vi "S4GUI_001.vi"() -> ()   [LabVIEW 2018] (continued)
        n876 = call-dynamic "Write PREV_FT.vi"("error in (no error)"=w1779, "PREV_FT"=w1776, "Interface in"=w1780) -> ("error out"=w1777:errorcluster, "Interface out"=w1778:refnum<class "Interface.lvclass">)  [unwired: 7 in]
        n877 = call-dynamic "Get CCD_Config.vi"("error in (no error)"=w1777, "Interface in"=w1778) -> ("error out"=w1817:errorcluster, "output cluster"=w1819:T24, "Interface out"=w1818:refnum<class "Interface.lvclass">)  [unwired: 7 in]
        n878 = Bundle By Name(cluster=w1819, "INITIAL_LINE"=w1816, "INITIAL_COLUMN"=w1815, "FINAL_LINE"=w1814, "FINAL_COLUMN"=w1813, "VBIN"=w1812, "HBIN"=w1811, "PREAMP"=w1810, "EM_GAIN"=w1809, "READOUT_RATE"=w1808, "SHUTTER_OPENING_TIME"=w1807, "SHUTTER_CLOSING_TIME"=w1806, "VERTICAL_SHIFT_SPEED"=w1805, "READ_MODE"=w1804, "VERTICAL_CLOCK_VOLTAGE"=w1803, "AD_CHANNEL"=w1802, "SHUTTER_MODE"=w1801, "SHUTTER_TTL"=w1800, "TRIGGER_MODE"=w1799, "FRAME_TRANSFER"=w1776, "ACQUISITION_MODE"=w1798, "EM_MODE"=w1797) -> (w1787:T24)
        n879 = call-dynamic "Set CCD_Config.vi"("error in (no error)"=w1817, "input cluster"=w1787, "Interface in"=w1818) -> ("error out"=w1822:errorcluster, "Interface out"=w1823:refnum<class "Interface.lvclass">)  [unwired: 7 in]
        n880 = Flatten To String(anything=w1787, error in (no error)=w1822) -> (data string=w1825:string, error out=w1824:errorcluster)  [unwired: 2 in, 1 out]
        n881 = call "Write flatted cluster.vi"("error in (no error)"=w1824, "flatted cluster"=w1825, "Interface in"=w1823) -> ("error out"=w1821:errorcluster, "Interface out"=w1820:refnum<class "Interface.lvclass">)  [unwired: 7 in]
        n882 = call-dynamic "Write Interface.vi"("error in (no error)"=w1821, "Interface.lvclass"=w1820, "Channel in"=w1838) -> ("error out"=w1792:errorcluster, "Channel out"=w1795:refnum<class "Channel.lvclass">)  [unwired: 7 in]
        n883 = call "Write section_name.vi"("error in (no error)"=w1792, "section_name"="CCD_ACS4", "Channel in"=w1795) -> ("error out"=w1791:errorcluster, "Channel out"=w1794:refnum<class "Channel.lvclass">)  [unwired: 7 in]
        n884 = call-dynamic "save config.vi"("error in (no error)"=w1791, "file config"="lastsaved.cfg", "Channel in"=w1794) -> ("error out"=w1790:errorcluster, "Channel out"=w1793:refnum<class "Channel.lvclass">)  [unwired: 7 in]
        n885 = call-dynamic "Read State Machine.vi"("error in (no error)"=w1790, "Device in"=w1793) -> ("error out"=w1832:errorcluster, "State Machine.lvclass"=w1834:refnum<class "State Machine.lvclass">, "Device out"=w1835:refnum<class "Channel.lvclass">)  [unwired: 7 in]
        n886 = call-dynamic "Write State.vi"("error in (no error)"=w1832, "State"=60, "State Machine in"=w1834) -> ("error out"=w1831:errorcluster, "State Machine out"=w1833:refnum<class "State Machine.lvclass">)  [unwired: 7 in]
        n887 = call-dynamic "Write State Machine.vi"("error in (no error)"=w1831, "State Machine.lvclass"=w1833, "Device in"=w1835) -> ("error out"=w1828:errorcluster, "Device out"=w1829:refnum<class "Channel.lvclass">)  [unwired: 7 in]
        n888 = call-dynamic "Write Channel.vi"("error in (no error)"=w1828, "Channel.lvclass"=w1829, "Acquisition in"=w1840) -> ("error out"=w1827:errorcluster, "Acquisition out"=w1826:refnum<class "Acquisition.lvclass">)  [unwired: 7 in]
        n889 = call-dynamic "Write AcquisitionD.vi"("error in (no error)"=w1827, "Acquisition.lvclass"=w1826, "S4ACS_GUI in"=w1842) -> ("error out"=w1781:errorcluster, "S4ACS_GUI out"=w1782:refnum<class "S4GUI.lvclass">)  [unwired: 7 in]
        n890 = call "Write cfg file.vi"("error in (no error)"=w1781, "cfg file"="lastsaved.cfg", "S4ACS_GUI in"=w1782) -> ("error out"=w1784:errorcluster, "S4ACS_GUI out"=w1785:refnum<class "S4GUI.lvclass">)  [unwired: 7 in]
      }
      event "Restore Default ch1": Value Change {
        n891 = event-data() -> ()  [unwired: 1 in, 6 out]
        n892 = call-dynamic "Read AcquisitionA.vi"("error in (no error)"=w1875, "S4ACS_GUI in"=w1876) -> ("error out"=w1871:errorcluster, "Acquisition.lvclass"=w1873:refnum<class "Acquisition.lvclass">, "S4ACS_GUI out"=w1874:refnum<class "S4GUI.lvclass">)  [unwired: 7 in]
        n893 = call-dynamic "Read Channel.vi"("error in (no error)"=w1871, "Acquisition in"=w1873) -> ("error out"=w1858:errorcluster, "Channel.lvclass"=w1860:refnum<class "Channel.lvclass">, "Acquisition out"=w1872:refnum<class "Acquisition.lvclass">)  [unwired: 7 in]
        n894 = call "Write section_name.vi"("error in (no error)"=w1858, "section_name"="CCD_ACS1", "Channel in"=w1860) -> ("error out"=w1857:errorcluster, "Channel out"=w1859:refnum<class "Channel.lvclass">)  [unwired: 7 in]
        n895 = call-dynamic "load config.vi"("error in (no error)"=w1857, "cfg file name"="default.cfg", "Channel in"=w1859) -> ("error out"=w1855:errorcluster, "Channel out"=w1856:refnum<class "Channel.lvclass">)  [unwired: 7 in]
        n896 = call-dynamic "Read State Machine.vi"("error in (no error)"=w1855, "Device in"=w1856) -> ("error out"=w1867:errorcluster, "State Machine.lvclass"=w1869:refnum<class "State Machine.lvclass">, "Device out"=w1870:refnum<class "Channel.lvclass">)  [unwired: 7 in]
        n897 = call-dynamic "Write State.vi"("error in (no error)"=w1867, "State"=60, "State Machine in"=w1869) -> ("error out"=w1866:errorcluster, "State Machine out"=w1868:refnum<class "State Machine.lvclass">)  [unwired: 7 in]
        n898 = call-dynamic "Write State Machine.vi"("error in (no error)"=w1866, "State Machine.lvclass"=w1868, "Device in"=w1870) -> ("error out"=w1851:errorcluster, "Device out"=w1847:refnum<class "Channel.lvclass">)  [unwired: 7 in]
        n899 = call "Write section_name.vi"("error in (no error)"=w1851, "section_name"="CCD_ACS1", "Channel in"=w1847) -> ("error out"=w1852:errorcluster, "Channel out"=w1846:refnum<class "Channel.lvclass">)  [unwired: 7 in]
        n900 = call-dynamic "save config.vi"("error in (no error)"=w1852, "file config"="lastsaved.cfg", "Channel in"=w1846) -> ("error out"=w1850:errorcluster, "Channel out"=w1845:refnum<class "Channel.lvclass">)  [unwired: 7 in]
        n901 = call-dynamic "Write Channel.vi"("error in (no error)"=w1850, "Channel.lvclass"=w1845, "Acquisition in"=w1872) -> ("error out"=w1864:errorcluster, "Acquisition out"=w1863:refnum<class "Acquisition.lvclass">)  [unwired: 7 in]
        n902 = call-dynamic "Write AcquisitionA.vi"("error in (no error)"=w1864, "Acquisition.lvclass"=w1863, "S4ACS_GUI in"=w1874) -> ("error out"=w1862:errorcluster, "S4ACS_GUI out"=w1853:refnum<class "S4GUI.lvclass">)  [unwired: 7 in]
      }
      event "Load Button": Value Change {
        n903 = event-data() -> ()  [unwired: 1 in, 6 out]
        n904 = call <vilib>:"Application Directory.vi"() -> ("Application Directory"=w1888:path)
        n905 = call "File Dialog"("start path"=w1888, "prompt"="Select file...", "button label"="Open", "default name"="lastsaved.cfg", "error in"=w1882, "pattern (all files)"="*.cfg") -> ("selected path"=w1880:path, "cancelled"=w1883:bool, "error out"=→"error out 2":errorcluster)  [unwired: 6 in, 1 out]
        "selected path" <- w1880
        n906 = Path To String(path=w1880) -> (string=w1879:string)
        n907 = Match Pattern(string=w1879, regular expression="SPARC4_GUI\\") -> (after substring=w1877:string)  [unwired: 1 in, 3 out]
        n908 = case shown="False" w1883 {
          tunnel: w1891 -> [w2000 w2002]
          tunnel: [w1916 w2002] -> w1890
          tunnel: [w1914 w2001] -> w1889
          tunnel: w1882 -> [w1913 w2001]
          tunnel: w1877 -> [w1912 _]
          frame False {
            n909 = call-dynamic "Read AcquisitionA.vi"("error in (no error)"=w1913, "S4ACS_GUI in"=w2000) -> ("error out"=w1996:errorcluster, "Acquisition.lvclass"=w1998:refnum<class "Acquisition.lvclass">, "S4ACS_GUI out"=w1999:refnum<class "S4GUI.lvclass">)  [unwired: 7 in]
            n910 = call-dynamic "Read Channel.vi"("error in (no error)"=w1996, "Acquisition in"=w1998) -> ("error out"=w1983:errorcluster, "Channel.lvclass"=w1985:refnum<class "Channel.lvclass">, "Acquisition out"=w1997:refnum<class "Acquisition.lvclass">)  [unwired: 7 in]
            n911 = call "Write section_name.vi"("error in (no error)"=w1983, "section_name"="CCD_ACS1", "Channel in"=w1985) -> ("error out"=w1982:errorcluster, "Channel out"=w1984:refnum<class "Channel.lvclass">)  [unwired: 7 in]
            n912 = call-dynamic "load config.vi"("error in (no error)"=w1982, "cfg file name"=w1912, "Channel in"=w1984) -> ("error out"=w1908:errorcluster, "Channel out"=w1910:refnum<class "Channel.lvclass">)  [unwired: 7 in]
            n913 = call-dynamic "save config.vi"("error in (no error)"=w1908, "file config"="lastsaved.cfg", "Channel in"=w1910) -> ("error out"=w1911:errorcluster, "Channel out"=w1909:refnum<class "Channel.lvclass">)  [unwired: 7 in]
            n914 = call-dynamic "Read State Machine.vi"("error in (no error)"=w1911, "Device in"=w1909) -> ("error out"=w1992:errorcluster, "State Machine.lvclass"=w1994:refnum<class "State Machine.lvclass">, "Device out"=w1995:refnum<class "Channel.lvclass">)  [unwired: 7 in]
            n915 = call-dynamic "Write State.vi"("error in (no error)"=w1992, "State"=60, "State Machine in"=w1994) -> ("error out"=w1991:errorcluster, "State Machine out"=w1993:refnum<class "State Machine.lvclass">)  [unwired: 7 in]
            n916 = call-dynamic "Write State Machine.vi"("error in (no error)"=w1991, "State Machine.lvclass"=w1993, "Device in"=w1995) -> ("error out"=w1988:errorcluster, "Device out"=w1989:refnum<class "Channel.lvclass">)  [unwired: 7 in]
            n917 = call-dynamic "Write Channel.vi"("error in (no error)"=w1988, "Channel.lvclass"=w1989, "Acquisition in"=w1997) -> ("error out"=w1987:errorcluster, "Acquisition out"=w1986:refnum<class "Acquisition.lvclass">)  [unwired: 7 in]
            n918 = call-dynamic "Write AcquisitionA.vi"("error in (no error)"=w1987, "Acquisition.lvclass"=w1986, "S4ACS_GUI in"=w1999) -> ("error out"=w1923:errorcluster, "S4ACS_GUI out"=w1922:refnum<class "S4GUI.lvclass">)  [unwired: 7 in]
            n919 = call "Read AcquisitionB.vi"("error in (no error)"=w1923, "S4ACS_GUI in"=w1922) -> ("error out"=w1965:errorcluster, "Acquisition.lvclass"=w1963:refnum<class "Acquisition.lvclass">, "S4ACS_GUI out"=w1962:refnum<class "S4GUI.lvclass">)  [unwired: 7 in]
            n920 = call-dynamic "Read Channel.vi"("error in (no error)"=w1965, "Acquisition in"=w1963) -> ("error out"=w1978:errorcluster, "Channel.lvclass"=w1976:refnum<class "Channel.lvclass">, "Acquisition out"=w1964:refnum<class "Acquisition.lvclass">)  [unwired: 7 in]
            n921 = call "Write section_name.vi"("error in (no error)"=w1978, "section_name"="CCD_ACS2", "Channel in"=w1976) -> ("error out"=w1979:errorcluster, "Channel out"=w1977:refnum<class "Channel.lvclass">)  [unwired: 7 in]
            n922 = call-dynamic "load config.vi"("error in (no error)"=w1979, "cfg file name"=w1912, "Channel in"=w1977) -> ("error out"=w1905:errorcluster, "Channel out"=w1903:refnum<class "Channel.lvclass">)  [unwired: 7 in]
            n923 = call-dynamic "save config.vi"("error in (no error)"=w1905, "file config"="lastsaved.cfg", "Channel in"=w1903) -> ("error out"=w1904:errorcluster, "Channel out"=w1902:refnum<class "Channel.lvclass">)  [unwired: 7 in]
            n924 = call-dynamic "Read State Machine.vi"("error in (no error)"=w1904, "Device in"=w1902) -> ("error out"=w1969:errorcluster, "State Machine.lvclass"=w1967:refnum<class "State Machine.lvclass">, "Device out"=w1966:refnum<class "Channel.lvclass">)  [unwired: 7 in]
            n925 = call-dynamic "Write State.vi"("error in (no error)"=w1969, "State"=60, "State Machine in"=w1967) -> ("error out"=w1970:errorcluster, "State Machine out"=w1968:refnum<class "State Machine.lvclass">)  [unwired: 7 in]
            n926 = call-dynamic "Write State Machine.vi"("error in (no error)"=w1970, "State Machine.lvclass"=w1968, "Device in"=w1966) -> ("error out"=w1973:errorcluster, "Device out"=w1972:refnum<class "Channel.lvclass">)  [unwired: 7 in]
            n927 = call-dynamic "Write Channel.vi"("error in (no error)"=w1973, "Channel.lvclass"=w1972, "Acquisition in"=w1964) -> ("error out"=w1974:errorcluster, "Acquisition out"=w1975:refnum<class "Acquisition.lvclass">)  [unwired: 7 in]
            n928 = call "Write AcquisitionB.vi"("error in (no error)"=w1974, "Acquisition.lvclass"=w1975, "S4ACS_GUI in"=w1962) -> ("error out"=w1921:errorcluster, "S4ACS_GUI out"=w1920:refnum<class "S4GUI.lvclass">)  [unwired: 7 in]
            n929 = call-dynamic "Read AcquisitionC.vi"("error in (no error)"=w1921, "S4ACS_GUI in"=w1920) -> ("error out"=w1958:errorcluster, "Acquisition.lvclass"=w1960:refnum<class "Acquisition.lvclass">, "S4ACS_GUI out"=w1961:refnum<class "S4GUI.lvclass">)  [unwired: 7 in]
            n930 = call-dynamic "Read Channel.vi"("error in (no error)"=w1958, "Acquisition in"=w1960) -> ("error out"=w1945:errorcluster, "Channel.lvclass"=w1947:refnum<class "Channel.lvclass">, "Acquisition out"=w1959:refnum<class "Acquisition.lvclass">)  [unwired: 7 in]
            n931 = call "Write section_name.vi"("error in (no error)"=w1945, "section_name"="CCD_ACS3", "Channel in"=w1947) -> ("error out"=w1944:errorcluster, "Channel out"=w1946:refnum<class "Channel.lvclass">)  [unwired: 7 in]
            n932 = call-dynamic "load config.vi"("error in (no error)"=w1944, "cfg file name"=w1912, "Channel in"=w1946) -> ("error out"=w1900:errorcluster, "Channel out"=w1898:refnum<class "Channel.lvclass">)  [unwired: 7 in]
            n933 = call-dynamic "save config.vi"("error in (no error)"=w1900, "file config"="lastsaved.cfg", "Channel in"=w1898) -> ("error out"=w1899:errorcluster, "Channel out"=w1897:refnum<class "Channel.lvclass">)  [unwired: 7 in]
            n934 = call-dynamic "Read State Machine.vi"("error in (no error)"=w1899, "Device in"=w1897) -> ("error out"=w1954:errorcluster, "State Machine.lvclass"=w1956:refnum<class "State Machine.lvclass">, "Device out"=w1957:refnum<class "Channel.lvclass">)  [unwired: 7 in]
            n935 = call-dynamic "Write State.vi"("error in (no error)"=w1954, "State"=60, "State Machine in"=w1956) -> ("error out"=w1953:errorcluster, "State Machine out"=w1955:refnum<class "State Machine.lvclass">)  [unwired: 7 in]
            n936 = call-dynamic "Write State Machine.vi"("error in (no error)"=w1953, "State Machine.lvclass"=w1955, "Device in"=w1957) -> ("error out"=w1950:errorcluster, "Device out"=w1951:refnum<class "Channel.lvclass">)  [unwired: 7 in]
            n937 = call-dynamic "Write Channel.vi"("error in (no error)"=w1950, "Channel.lvclass"=w1951, "Acquisition in"=w1959) -> ("error out"=w1949:errorcluster, "Acquisition out"=w1948:refnum<class "Acquisition.lvclass">)  [unwired: 7 in]
            n938 = call-dynamic "Write AcquisitionC.vi"("error in (no error)"=w1949, "Acquisition.lvclass"=w1948, "S4ACS_GUI in"=w1961) -> ("error out"=w1919:errorcluster, "S4ACS_GUI out"=w1918:refnum<class "S4GUI.lvclass">)  [unwired: 7 in]
            n939 = call-dynamic "Read AcquisitionD.vi"("error in (no error)"=w1919, "S4ACS_GUI in"=w1918) -> ("error out"=w1927:errorcluster, "Acquisition.lvclass"=w1925:refnum<class "Acquisition.lvclass">, "S4ACS_GUI out"=w1924:refnum<class "S4GUI.lvclass">)  [unwired: 7 in]
            n940 = call-dynamic "Read Channel.vi"("error in (no error)"=w1927, "Acquisition in"=w1925) -> ("error out"=w1940:errorcluster, "Channel.lvclass"=w1938:refnum<class "Channel.lvclass">, "Acquisition out"=w1926:refnum<class "Acquisition.lvclass">)  [unwired: 7 in]
            n941 = call "Write section_name.vi"("error in (no error)"=w1940, "section_name"="CCD_ACS4", "Channel in"=w1938) -> ("error out"=w1941:errorcluster, "Channel out"=w1939:refnum<class "Channel.lvclass">)  [unwired: 7 in]
            n942 = call-dynamic "load config.vi"("error in (no error)"=w1941, "cfg file name"=w1912, "Channel in"=w1939) -> ("error out"=w1896:errorcluster, "Channel out"=w1894:refnum<class "Channel.lvclass">)  [unwired: 7 in]
            n943 = call-dynamic "save config.vi"("error in (no error)"=w1896, "file config"="lastsaved.cfg", "Channel in"=w1894) -> ("error out"=w1895:errorcluster, "Channel out"=w1893:refnum<class "Channel.lvclass">)  [unwired: 7 in]
            n944 = call-dynamic "Read State Machine.vi"("error in (no error)"=w1895, "Device in"=w1893) -> ("error out"=w1931:errorcluster, "State Machine.lvclass"=w1929:refnum<class "State Machine.lvclass">, "Device out"=w1928:refnum<class "Channel.lvclass">)  [unwired: 7 in]
            n945 = call-dynamic "Write State.vi"("error in (no error)"=w1931, "State"=60, "State Machine in"=w1929) -> ("error out"=w1932:errorcluster, "State Machine out"=w1930:refnum<class "State Machine.lvclass">)  [unwired: 7 in]
            n946 = call-dynamic "Write State Machine.vi"("error in (no error)"=w1932, "State Machine.lvclass"=w1930, "Device in"=w1928) -> ("error out"=w1935:errorcluster, "Device out"=w1934:refnum<class "Channel.lvclass">)  [unwired: 7 in]
            n947 = call-dynamic "Write Channel.vi"("error in (no error)"=w1935, "Channel.lvclass"=w1934, "Acquisition in"=w1926) -> ("error out"=w1936:errorcluster, "Acquisition out"=w1937:refnum<class "Acquisition.lvclass">)  [unwired: 7 in]
            n948 = call-dynamic "Write AcquisitionD.vi"("error in (no error)"=w1936, "Acquisition.lvclass"=w1937, "S4ACS_GUI in"=w1924) -> ("error out"=w1915:errorcluster, "S4ACS_GUI out"=w1917:refnum<class "S4GUI.lvclass">)  [unwired: 7 in]
            n949 = call "Write cfg file.vi"("error in (no error)"=w1915, "cfg file"=w1912, "S4ACS_GUI in"=w1917) -> ("error out"=w1914:errorcluster, "S4ACS_GUI out"=w1916:refnum<class "S4GUI.lvclass">)  [unwired: 7 in]
          }
          frame True {
          }
        }
      }
      event "Save As Button": Value Change {
        n950 = event-data() -> ()  [unwired: 1 in, 6 out]
        n951 = call <vilib>:"Application Directory.vi"() -> ("Application Directory"=w2014:path)
        n952 = call "File Dialog2"("start path"=w2014, "prompt"="Select file...", "button label"="Save", "default name"="lastsaved.cfg", "error in"=w2008, "pattern (all files)"="*.cfg") -> ("selected path"=w2006:path, "cancelled"=w2009:bool, "error out"=→"error out 3":errorcluster)  [unwired: 6 in, 1 out]
        n953 = Path To String(path=w2006) -> (string=w2005:string)
        n954 = Match Pattern(string=w2005, regular expression="SPARC4_GUI\\") -> (after substring=w2003:string)  [unwired: 1 in, 3 out]
        n955 = case shown="False" w2009 {
          tunnel: w2017 -> [w2082 w2084]
          tunnel: [w2030 w2084] -> w2016
          tunnel: [w2028 w2083] -> w2015
          tunnel: w2008 -> [w2027 w2083]
          tunnel: w2003 -> [w2026 _]
          frame False {
            n956 = call-dynamic "Read AcquisitionA.vi"("error in (no error)"=w2027, "S4ACS_GUI in"=w2082) -> ("error out"=w2078:errorcluster, "Acquisition.lvclass"=w2080:refnum<class "Acquisition.lvclass">, "S4ACS_GUI out"=w2081:refnum<class "S4GUI.lvclass">)  [unwired: 7 in]
            n957 = call-dynamic "Read Channel.vi"("error in (no error)"=w2078, "Acquisition in"=w2080) -> ("error out"=w2073:errorcluster, "Channel.lvclass"=w2075:refnum<class "Channel.lvclass">, "Acquisition out"=w2079:refnum<class "Acquisition.lvclass">)  [unwired: 7 in]
            n958 = call "Write section_name.vi"("error in (no error)"=w2073, "section_name"="CCD_ACS1", "Channel in"=w2075) -> ("error out"=w2072:errorcluster, "Channel out"=w2074:refnum<class "Channel.lvclass">)  [unwired: 7 in]
            n959 = call-dynamic "save config.vi"("error in (no error)"=w2072, "file config"=w2026, "Channel in"=w2074) -> ("error out"=w2024:errorcluster, "Channel out"=w2025:refnum<class "Channel.lvclass">)  [unwired: 7 in]
            n960 = call-dynamic "Write Channel.vi"("error in (no error)"=w2024, "Channel.lvclass"=w2025, "Acquisition in"=w2079) -> ("error out"=w2077:errorcluster, "Acquisition out"=w2076:refnum<class "Acquisition.lvclass">)  [unwired: 7 in]
            n961 = call-dynamic "Write AcquisitionA.vi"("error in (no error)"=w2077, "Acquisition.lvclass"=w2076, "S4ACS_GUI in"=w2081) -> ("error out"=w2037:errorcluster, "S4ACS_GUI out"=w2036:refnum<class "S4GUI.lvclass">)  [unwired: 7 in]
            n962 = call "Read AcquisitionB.vi"("error in (no error)"=w2037, "S4ACS_GUI in"=w2036) -> ("error out"=w2063:errorcluster, "Acquisition.lvclass"=w2061:refnum<class "Acquisition.lvclass">, "S4ACS_GUI out"=w2060:refnum<class "S4GUI.lvclass">)  [unwired: 7 in]
            n963 = call-dynamic "Read Channel.vi"("error in (no error)"=w2063, "Acquisition in"=w2061) -> ("error out"=w2068:errorcluster, "Channel.lvclass"=w2066:refnum<class "Channel.lvclass">, "Acquisition out"=w2062:refnum<class "Acquisition.lvclass">)  [unwired: 7 in]
            n964 = call "Write section_name.vi"("error in (no error)"=w2068, "section_name"="CCD_ACS2", "Channel in"=w2066) -> ("error out"=w2069:errorcluster, "Channel out"=w2067:refnum<class "Channel.lvclass">)  [unwired: 7 in]
            n965 = call-dynamic "save config.vi"("error in (no error)"=w2069, "file config"=w2026, "Channel in"=w2067) -> ("error out"=w2018:errorcluster, "Channel out"=w2019:refnum<class "Channel.lvclass">)  [unwired: 7 in]
            n966 = call-dynamic "Write Channel.vi"("error in (no error)"=w2018, "Channel.lvclass"=w2019, "Acquisition in"=w2062) -> ("error out"=w2064:errorcluster, "Acquisition out"=w2065:refnum<class "Acquisition.lvclass">)  [unwired: 7 in]
            n967 = call "Write AcquisitionB.vi"("error in (no error)"=w2064, "Acquisition.lvclass"=w2065, "S4ACS_GUI in"=w2060) -> ("error out"=w2035:errorcluster, "S4ACS_GUI out"=w2034:refnum<class "S4GUI.lvclass">)  [unwired: 7 in]
            n968 = call-dynamic "Read AcquisitionC.vi"("error in (no error)"=w2035, "S4ACS_GUI in"=w2034) -> ("error out"=w2056:errorcluster, "Acquisition.lvclass"=w2058:refnum<class "Acquisition.lvclass">, "S4ACS_GUI out"=w2059:refnum<class "S4GUI.lvclass">)  [unwired: 7 in]
            n969 = call-dynamic "Read Channel.vi"("error in (no error)"=w2056, "Acquisition in"=w2058) -> ("error out"=w2051:errorcluster, "Channel.lvclass"=w2053:refnum<class "Channel.lvclass">, "Acquisition out"=w2057:refnum<class "Acquisition.lvclass">)  [unwired: 7 in]
            n970 = call "Write section_name.vi"("error in (no error)"=w2051, "section_name"="CCD_ACS3", "Channel in"=w2053) -> ("error out"=w2050:errorcluster, "Channel out"=w2052:refnum<class "Channel.lvclass">)  [unwired: 7 in]
            n971 = call-dynamic "save config.vi"("error in (no error)"=w2050, "file config"=w2026, "Channel in"=w2052) -> ("error out"=w2020:errorcluster, "Channel out"=w2021:refnum<class "Channel.lvclass">)  [unwired: 7 in]
            n972 = call-dynamic "Write Channel.vi"("error in (no error)"=w2020, "Channel.lvclass"=w2021, "Acquisition in"=w2057) -> ("error out"=w2055:errorcluster, "Acquisition out"=w2054:refnum<class "Acquisition.lvclass">)  [unwired: 7 in]
            n973 = call-dynamic "Write AcquisitionC.vi"("error in (no error)"=w2055, "Acquisition.lvclass"=w2054, "S4ACS_GUI in"=w2059) -> ("error out"=w2033:errorcluster, "S4ACS_GUI out"=w2032:refnum<class "S4GUI.lvclass">)  [unwired: 7 in]
            n974 = call-dynamic "Read AcquisitionD.vi"("error in (no error)"=w2033, "S4ACS_GUI in"=w2032) -> ("error out"=w2041:errorcluster, "Acquisition.lvclass"=w2039:refnum<class "Acquisition.lvclass">, "S4ACS_GUI out"=w2038:refnum<class "S4GUI.lvclass">)  [unwired: 7 in]
            n975 = call-dynamic "Read Channel.vi"("error in (no error)"=w2041, "Acquisition in"=w2039) -> ("error out"=w2046:errorcluster, "Channel.lvclass"=w2044:refnum<class "Channel.lvclass">, "Acquisition out"=w2040:refnum<class "Acquisition.lvclass">)  [unwired: 7 in]
            n976 = call "Write section_name.vi"("error in (no error)"=w2046, "section_name"="CCD_ACS4", "Channel in"=w2044) -> ("error out"=w2047:errorcluster, "Channel out"=w2045:refnum<class "Channel.lvclass">)  [unwired: 7 in]
            n977 = call-dynamic "save config.vi"("error in (no error)"=w2047, "file config"=w2026, "Channel in"=w2045) -> ("error out"=w2022:errorcluster, "Channel out"=w2023:refnum<class "Channel.lvclass">)  [unwired: 7 in]
            n978 = call-dynamic "Write Channel.vi"("error in (no error)"=w2022, "Channel.lvclass"=w2023, "Acquisition in"=w2040) -> ("error out"=w2042:errorcluster, "Acquisition out"=w2043:refnum<class "Acquisition.lvclass">)  [unwired: 7 in]
            n979 = call-dynamic "Write AcquisitionD.vi"("error in (no error)"=w2042, "Acquisition.lvclass"=w2043, "S4ACS_GUI in"=w2038) -> ("error out"=w2029:errorcluster, "S4ACS_GUI out"=w2031:refnum<class "S4GUI.lvclass">)  [unwired: 7 in]
            n980 = call "Write cfg file.vi"("error in (no error)"=w2029, "cfg file"=w2026, "S4ACS_GUI in"=w2031) -> ("error out"=w2028:errorcluster, "S4ACS_GUI out"=w2030:refnum<class "S4GUI.lvclass">)  [unwired: 7 in]
          }
          frame True {
          }
        }
      }
      event "Load Default Button": Value Change {
        w2105 = "default.cfg" ("cfg file name")
        n981 = event-data() -> ()  [unwired: 1 in, 6 out]
        n982 = call-dynamic "Read AcquisitionA.vi"("error in (no error)"=w2195, "S4ACS_GUI in"=w2196) -> ("error out"=w2191:errorcluster, "Acquisition.lvclass"=w2193:refnum<class "Acquisition.lvclass">, "S4ACS_GUI out"=w2194:refnum<class "S4GUI.lvclass">)  [unwired: 7 in]
        n983 = call-dynamic "Read Channel.vi"("error in (no error)"=w2191, "Acquisition in"=w2193) -> ("error out"=w2178:errorcluster, "Channel.lvclass"=w2180:refnum<class "Channel.lvclass">, "Acquisition out"=w2192:refnum<class "Acquisition.lvclass">)  [unwired: 7 in]
        n984 = call "Write section_name.vi"("error in (no error)"=w2178, "section_name"="CCD_ACS1", "Channel in"=w2180) -> ("error out"=w2177:errorcluster, "Channel out"=w2179:refnum<class "Channel.lvclass">)  [unwired: 7 in]
        n985 = call-dynamic "load config.vi"("error in (no error)"=w2177, "cfg file name"=w2105, "Channel in"=w2179) -> ("error out"=w2102:errorcluster, "Channel out"=w2104:refnum<class "Channel.lvclass">)  [unwired: 7 in]
        n986 = call-dynamic "save config.vi"("error in (no error)"=w2102, "file config"="lastsaved.cfg", "Channel in"=w2104) -> ("error out"=w2101:errorcluster, "Channel out"=w2103:refnum<class "Channel.lvclass">)  [unwired: 7 in]
        n987 = call-dynamic "Read State Machine.vi"("error in (no error)"=w2101, "Device in"=w2103) -> ("error out"=w2187:errorcluster, "State Machine.lvclass"=w2189:refnum<class "State Machine.lvclass">, "Device out"=w2190:refnum<class "Channel.lvclass">)  [unwired: 7 in]
        n988 = call-dynamic "Write State.vi"("error in (no error)"=w2187, "State"=60, "State Machine in"=w2189) -> ("error out"=w2186:errorcluster, "State Machine out"=w2188:refnum<class "State Machine.lvclass">)  [unwired: 7 in]
        n989 = call-dynamic "Write State Machine.vi"("error in (no error)"=w2186, "State Machine.lvclass"=w2188, "Device in"=w2190) -> ("error out"=w2183:errorcluster, "Device out"=w2184:refnum<class "Channel.lvclass">)  [unwired: 7 in]
        n990 = call-dynamic "Write Channel.vi"("error in (no error)"=w2183, "Channel.lvclass"=w2184, "Acquisition in"=w2192) -> ("error out"=w2182:errorcluster, "Acquisition out"=w2181:refnum<class "Acquisition.lvclass">)  [unwired: 7 in]
        n991 = call-dynamic "Write AcquisitionA.vi"("error in (no error)"=w2182, "Acquisition.lvclass"=w2181, "S4ACS_GUI in"=w2194) -> ("error out"=w2115:errorcluster, "S4ACS_GUI out"=w2114:refnum<class "S4GUI.lvclass">)  [unwired: 7 in]
        n992 = call "Read AcquisitionB.vi"("error in (no error)"=w2115, "S4ACS_GUI in"=w2114) -> ("error out"=w2159:errorcluster, "Acquisition.lvclass"=w2157:refnum<class "Acquisition.lvclass">, "S4ACS_GUI out"=w2156:refnum<class "S4GUI.lvclass">)  [unwired: 7 in]
        n993 = call-dynamic "Read Channel.vi"("error in (no error)"=w2159, "Acquisition in"=w2157) -> ("error out"=w2173:errorcluster, "Channel.lvclass"=w2171:refnum<class "Channel.lvclass">, "Acquisition out"=w2158:refnum<class "Acquisition.lvclass">)  [unwired: 7 in]
        n994 = call "Write section_name.vi"("error in (no error)"=w2173, "section_name"="CCD_ACS2", "Channel in"=w2171) -> ("error out"=w2174:errorcluster, "Channel out"=w2172:refnum<class "Channel.lvclass">)  [unwired: 7 in]
        n995 = call-dynamic "load config.vi"("error in (no error)"=w2174, "cfg file name"="default.cfg", "Channel in"=w2172) -> ("error out"=w2098:errorcluster, "Channel out"=w2096:refnum<class "Channel.lvclass">)  [unwired: 7 in]
        n996 = call-dynamic "save config.vi"("error in (no error)"=w2098, "file config"="lastsaved.cfg", "Channel in"=w2096) -> ("error out"=w2097:errorcluster, "Channel out"=w2095:refnum<class "Channel.lvclass">)  [unwired: 7 in]
        n997 = call-dynamic "Read State Machine.vi"("error in (no error)"=w2097, "Device in"=w2095) -> ("error out"=w2163:errorcluster, "State Machine.lvclass"=w2161:refnum<class "State Machine.lvclass">, "Device out"=w2160:refnum<class "Channel.lvclass">)  [unwired: 7 in]
        n998 = call-dynamic "Write State.vi"("error in (no error)"=w2163, "State"=60, "State Machine in"=w2161) -> ("error out"=w2164:errorcluster, "State Machine out"=w2162:refnum<class "State Machine.lvclass">)  [unwired: 7 in]
        n999 = call-dynamic "Write State Machine.vi"("error in (no error)"=w2164, "State Machine.lvclass"=w2162, "Device in"=w2160) -> ("error out"=w2167:errorcluster, "Device out"=w2166:refnum<class "Channel.lvclass">)  [unwired: 7 in]
        n1000 = call-dynamic "Write Channel.vi"("error in (no error)"=w2167, "Channel.lvclass"=w2166, "Acquisition in"=w2158) -> ("error out"=w2168:errorcluster, "Acquisition out"=w2169:refnum<class "Acquisition.lvclass">)  [unwired: 7 in]
        n1001 = call "Write AcquisitionB.vi"("error in (no error)"=w2168, "Acquisition.lvclass"=w2169, "S4ACS_GUI in"=w2156) -> ("error out"=w2113:errorcluster, "S4ACS_GUI out"=w2112:refnum<class "S4GUI.lvclass">)  [unwired: 7 in]
        n1002 = call-dynamic "Read AcquisitionC.vi"("error in (no error)"=w2113, "S4ACS_GUI in"=w2112) -> ("error out"=w2152:errorcluster, "Acquisition.lvclass"=w2154:refnum<class "Acquisition.lvclass">, "S4ACS_GUI out"=w2155:refnum<class "S4GUI.lvclass">)  [unwired: 7 in]
        n1003 = call-dynamic "Read Channel.vi"("error in (no error)"=w2152, "Acquisition in"=w2154) -> ("error out"=w2138:errorcluster, "Channel.lvclass"=w2140:refnum<class "Channel.lvclass">, "Acquisition out"=w2153:refnum<class "Acquisition.lvclass">)  [unwired: 7 in]
        n1004 = call "Write section_name.vi"("error in (no error)"=w2138, "section_name"="CCD_ACS3", "Channel in"=w2140) -> ("error out"=w2137:errorcluster, "Channel out"=w2139:refnum<class "Channel.lvclass">)  [unwired: 7 in]
        n1005 = call-dynamic "load config.vi"("error in (no error)"=w2137, "cfg file name"="default.cfg", "Channel in"=w2139) -> ("error out"=w2092:errorcluster, "Channel out"=w2093:refnum<class "Channel.lvclass">)  [unwired: 7 in]
        n1006 = call-dynamic "save config.vi"("error in (no error)"=w2092, "file config"="lastsaved.cfg", "Channel in"=w2093) -> ("error out"=w2090:errorcluster, "Channel out"=w2091:refnum<class "Channel.lvclass">)  [unwired: 7 in]
        n1007 = call-dynamic "Read State Machine.vi"("error in (no error)"=w2090, "Device in"=w2091) -> ("error out"=w2148:errorcluster, "State Machine.lvclass"=w2150:refnum<class "State Machine.lvclass">, "Device out"=w2151:refnum<class "Channel.lvclass">)  [unwired: 7 in]
        n1008 = call-dynamic "Write State.vi"("error in (no error)"=w2148, "State"=60, "State Machine in"=w2150) -> ("error out"=w2147:errorcluster, "State Machine out"=w2149:refnum<class "State Machine.lvclass">)  [unwired: 7 in]
        n1009 = call-dynamic "Write State Machine.vi"("error in (no error)"=w2147, "State Machine.lvclass"=w2149, "Device in"=w2151) -> ("error out"=w2144:errorcluster, "Device out"=w2145:refnum<class "Channel.lvclass">)  [unwired: 7 in]
        n1010 = call-dynamic "Write Channel.vi"("error in (no error)"=w2144, "Channel.lvclass"=w2145, "Acquisition in"=w2153) -> ("error out"=w2143:errorcluster, "Acquisition out"=w2142:refnum<class "Acquisition.lvclass">)  [unwired: 7 in]
        n1011 = call-dynamic "Write AcquisitionC.vi"("error in (no error)"=w2143, "Acquisition.lvclass"=w2142, "S4ACS_GUI in"=w2155) -> ("error out"=w2111:errorcluster, "S4ACS_GUI out"=w2110:refnum<class "S4GUI.lvclass">)  [unwired: 7 in]
        n1012 = call-dynamic "Read AcquisitionD.vi"("error in (no error)"=w2111, "S4ACS_GUI in"=w2110) -> ("error out"=w2119:errorcluster, "Acquisition.lvclass"=w2117:refnum<class "Acquisition.lvclass">, "S4ACS_GUI out"=w2116:refnum<class "S4GUI.lvclass">)  [unwired: 7 in]
        n1013 = call-dynamic "Read Channel.vi"("error in (no error)"=w2119, "Acquisition in"=w2117) -> ("error out"=w2133:errorcluster, "Channel.lvclass"=w2131:refnum<class "Channel.lvclass">, "Acquisition out"=w2118:refnum<class "Acquisition.lvclass">)  [unwired: 7 in]
        n1014 = call "Write section_name.vi"("error in (no error)"=w2133, "section_name"="CCD_ACS4", "Channel in"=w2131) -> ("error out"=w2134:errorcluster, "Channel out"=w2132:refnum<class "Channel.lvclass">)  [unwired: 7 in]
        n1015 = call-dynamic "load config.vi"("error in (no error)"=w2134, "cfg file name"="default.cfg", "Channel in"=w2132) -> ("error out"=w2088:errorcluster, "Channel out"=w2087:refnum<class "Channel.lvclass">)  [unwired: 7 in]
        n1016 = call-dynamic "save config.vi"("error in (no error)"=w2088, "file config"="lastsaved.cfg", "Channel in"=w2087) -> ("error out"=w2085:errorcluster, "Channel out"=w2086:refnum<class "Channel.lvclass">)  [unwired: 7 in]
        n1017 = call-dynamic "Read State Machine.vi"("error in (no error)"=w2085, "Device in"=w2086) -> ("error out"=w2123:errorcluster, "State Machine.lvclass"=w2121:refnum<class "State Machine.lvclass">, "Device out"=w2120:refnum<class "Channel.lvclass">)  [unwired: 7 in]
        n1018 = call-dynamic "Write State.vi"("error in (no error)"=w2123, "State"=60, "State Machine in"=w2121) -> ("error out"=w2124:errorcluster, "State Machine out"=w2122:refnum<class "State Machine.lvclass">)  [unwired: 7 in]
        n1019 = call-dynamic "Write State Machine.vi"("error in (no error)"=w2124, "State Machine.lvclass"=w2122, "Device in"=w2120) -> ("error out"=w2127:errorcluster, "Device out"=w2126:refnum<class "Channel.lvclass">)  [unwired: 7 in]
        n1020 = call-dynamic "Write Channel.vi"("error in (no error)"=w2127, "Channel.lvclass"=w2126, "Acquisition in"=w2118) -> ("error out"=w2128:errorcluster, "Acquisition out"=w2129:refnum<class "Acquisition.lvclass">)  [unwired: 7 in]
        n1021 = call-dynamic "Write AcquisitionD.vi"("error in (no error)"=w2128, "Acquisition.lvclass"=w2129, "S4ACS_GUI in"=w2116) -> ("error out"=w2107:errorcluster, "S4ACS_GUI out"=w2109:refnum<class "S4GUI.lvclass">)  [unwired: 7 in]
        n1022 = call "Write cfg file.vi"("error in (no error)"=w2107, "cfg file"=w2105, "S4ACS_GUI in"=w2109) -> ("error out"=w2106:errorcluster, "S4ACS_GUI out"=w2108:refnum<class "S4GUI.lvclass">)  [unwired: 7 in]
      }
      event "Restore Default ch2": Value Change {
        n1023 = event-data() -> ()  [unwired: 1 in, 6 out]
        n1024 = call "Read AcquisitionB.vi"("error in (no error)"=w2227, "S4ACS_GUI in"=w2228) -> ("error out"=w2223:errorcluster, "Acquisition.lvclass"=w2225:refnum<class "Acquisition.lvclass">, "S4ACS_GUI out"=w2226:refnum<class "S4GUI.lvclass">)  [unwired: 7 in]
        n1025 = call-dynamic "Read Channel.vi"("error in (no error)"=w2223, "Acquisition in"=w2225) -> ("error out"=w2210:errorcluster, "Channel.lvclass"=w2212:refnum<class "Channel.lvclass">, "Acquisition out"=w2224:refnum<class "Acquisition.lvclass">)  [unwired: 7 in]
        n1026 = call "Write section_name.vi"("error in (no error)"=w2210, "section_name"="CCD_ACS2", "Channel in"=w2212) -> ("error out"=w2209:errorcluster, "Channel out"=w2211:refnum<class "Channel.lvclass">)  [unwired: 7 in]
        n1027 = call-dynamic "load config.vi"("error in (no error)"=w2209, "cfg file name"="default.cfg", "Channel in"=w2211) -> ("error out"=w2207:errorcluster, "Channel out"=w2208:refnum<class "Channel.lvclass">)  [unwired: 7 in]
        n1028 = call-dynamic "Read State Machine.vi"("error in (no error)"=w2207, "Device in"=w2208) -> ("error out"=w2219:errorcluster, "State Machine.lvclass"=w2221:refnum<class "State Machine.lvclass">, "Device out"=w2222:refnum<class "Channel.lvclass">)  [unwired: 7 in]
        n1029 = call-dynamic "Write State.vi"("error in (no error)"=w2219, "State"=60, "State Machine in"=w2221) -> ("error out"=w2218:errorcluster, "State Machine out"=w2220:refnum<class "State Machine.lvclass">)  [unwired: 7 in]
        n1030 = call-dynamic "Write State Machine.vi"("error in (no error)"=w2218, "State Machine.lvclass"=w2220, "Device in"=w2222) -> ("error out"=w2203:errorcluster, "Device out"=w2200:refnum<class "Channel.lvclass">)  [unwired: 7 in]
        n1031 = call "Write section_name.vi"("error in (no error)"=w2203, "section_name"="CCD_ACS2", "Channel in"=w2200) -> ("error out"=w2204:errorcluster, "Channel out"=w2199:refnum<class "Channel.lvclass">)  [unwired: 7 in]
        n1032 = call-dynamic "save config.vi"("error in (no error)"=w2204, "file config"="lastsaved.cfg", "Channel in"=w2199) -> ("error out"=w2202:errorcluster, "Channel out"=w2198:refnum<class "Channel.lvclass">)  [unwired: 7 in]
        n1033 = call-dynamic "Write Channel.vi"("error in (no error)"=w2202, "Channel.lvclass"=w2198, "Acquisition in"=w2224) -> ("error out"=w2216:errorcluster, "Acquisition out"=w2215:refnum<class "Acquisition.lvclass">)  [unwired: 7 in]
        n1034 = call "Write AcquisitionB.vi"("error in (no error)"=w2216, "Acquisition.lvclass"=w2215, "S4ACS_GUI in"=w2226) -> ("error out"=w2214:errorcluster, "S4ACS_GUI out"=w2205:refnum<class "S4GUI.lvclass">)  [unwired: 7 in]
      }
      event "Restore Default ch3": Value Change {
        n1035 = event-data() -> ()  [unwired: 1 in, 6 out]
        n1036 = call-dynamic "Read AcquisitionC.vi"("error in (no error)"=w2259, "S4ACS_GUI in"=w2260) -> ("error out"=w2255:errorcluster, "Acquisition.lvclass"=w2257:refnum<class "Acquisition.lvclass">, "S4ACS_GUI out"=w2258:refnum<class "S4GUI.lvclass">)  [unwired: 7 in]
        n1037 = call-dynamic "Read Channel.vi"("error in (no error)"=w2255, "Acquisition in"=w2257) -> ("error out"=w2242:errorcluster, "Channel.lvclass"=w2244:refnum<class "Channel.lvclass">, "Acquisition out"=w2256:refnum<class "Acquisition.lvclass">)  [unwired: 7 in]
        n1038 = call "Write section_name.vi"("error in (no error)"=w2242, "section_name"="CCD_ACS3", "Channel in"=w2244) -> ("error out"=w2241:errorcluster, "Channel out"=w2243:refnum<class "Channel.lvclass">)  [unwired: 7 in]
        n1039 = call-dynamic "load config.vi"("error in (no error)"=w2241, "cfg file name"="default.cfg", "Channel in"=w2243) -> ("error out"=w2239:errorcluster, "Channel out"=w2240:refnum<class "Channel.lvclass">)  [unwired: 7 in]
        n1040 = call-dynamic "Read State Machine.vi"("error in (no error)"=w2239, "Device in"=w2240) -> ("error out"=w2251:errorcluster, "State Machine.lvclass"=w2253:refnum<class "State Machine.lvclass">, "Device out"=w2254:refnum<class "Channel.lvclass">)  [unwired: 7 in]
        n1041 = call-dynamic "Write State.vi"("error in (no error)"=w2251, "State"=60, "State Machine in"=w2253) -> ("error out"=w2250:errorcluster, "State Machine out"=w2252:refnum<class "State Machine.lvclass">)  [unwired: 7 in]
        n1042 = call-dynamic "Write State Machine.vi"("error in (no error)"=w2250, "State Machine.lvclass"=w2252, "Device in"=w2254) -> ("error out"=w2230:errorcluster, "Device out"=w2232:refnum<class "Channel.lvclass">)  [unwired: 7 in]
        n1043 = call "Write section_name.vi"("error in (no error)"=w2230, "section_name"="CCD_ACS3", "Channel in"=w2232) -> ("error out"=w2236:errorcluster, "Channel out"=w2231:refnum<class "Channel.lvclass">)  [unwired: 7 in]
        n1044 = call-dynamic "save config.vi"("error in (no error)"=w2236, "file config"="lastsaved.cfg", "Channel in"=w2231) -> ("error out"=w2229:errorcluster, "Channel out"=w2233:refnum<class "Channel.lvclass">)  [unwired: 7 in]
        n1045 = call-dynamic "Write Channel.vi"("error in (no error)"=w2229, "Channel.lvclass"=w2233, "Acquisition in"=w2256) -> ("error out"=w2248:errorcluster, "Acquisition out"=w2247:refnum<class "Acquisition.lvclass">)  [unwired: 7 in]
        n1046 = call-dynamic "Write AcquisitionC.vi"("error in (no error)"=w2248, "Acquisition.lvclass"=w2247, "S4ACS_GUI in"=w2258) -> ("error out"=w2246:errorcluster, "S4ACS_GUI out"=w2237:refnum<class "S4GUI.lvclass">)  [unwired: 7 in]
      }
      event "Restore Default ch4": Value Change {
        n1047 = event-data() -> ()  [unwired: 1 in, 6 out]
        n1048 = call-dynamic "Read AcquisitionD.vi"("error in (no error)"=w2291, "S4ACS_GUI in"=w2292) -> ("error out"=w2287:errorcluster, "Acquisition.lvclass"=w2289:refnum<class "Acquisition.lvclass">, "S4ACS_GUI out"=w2290:refnum<class "S4GUI.lvclass">)  [unwired: 7 in]
        n1049 = call-dynamic "Read Channel.vi"("error in (no error)"=w2287, "Acquisition in"=w2289) -> ("error out"=w2274:errorcluster, "Channel.lvclass"=w2276:refnum<class "Channel.lvclass">, "Acquisition out"=w2288:refnum<class "Acquisition.lvclass">)  [unwired: 7 in]
        n1050 = call "Write section_name.vi"("error in (no error)"=w2274, "section_name"="CCD_ACS4", "Channel in"=w2276) -> ("error out"=w2273:errorcluster, "Channel out"=w2275:refnum<class "Channel.lvclass">)  [unwired: 7 in]
        n1051 = call-dynamic "load config.vi"("error in (no error)"=w2273, "cfg file name"="default.cfg", "Channel in"=w2275) -> ("error out"=w2271:errorcluster, "Channel out"=w2272:refnum<class "Channel.lvclass">)  [unwired: 7 in]
        n1052 = call-dynamic "Read State Machine.vi"("error in (no error)"=w2271, "Device in"=w2272) -> ("error out"=w2283:errorcluster, "State Machine.lvclass"=w2285:refnum<class "State Machine.lvclass">, "Device out"=w2286:refnum<class "Channel.lvclass">)  [unwired: 7 in]
        n1053 = call-dynamic "Write State.vi"("error in (no error)"=w2283, "State"=60, "State Machine in"=w2285) -> ("error out"=w2282:errorcluster, "State Machine out"=w2284:refnum<class "State Machine.lvclass">)  [unwired: 7 in]
        n1054 = call-dynamic "Write State Machine.vi"("error in (no error)"=w2282, "State Machine.lvclass"=w2284, "Device in"=w2286) -> ("error out"=w2262:errorcluster, "Device out"=w2265:refnum<class "Channel.lvclass">)  [unwired: 7 in]
        n1055 = call "Write section_name.vi"("error in (no error)"=w2262, "section_name"="CCD_ACS4", "Channel in"=w2265) -> ("error out"=w2268:errorcluster, "Channel out"=w2264:refnum<class "Channel.lvclass">)  [unwired: 7 in]
        n1056 = call-dynamic "save config.vi"("error in (no error)"=w2268, "file config"="lastsaved.cfg", "Channel in"=w2264) -> ("error out"=w2261:errorcluster, "Channel out"=w2263:refnum<class "Channel.lvclass">)  [unwired: 7 in]
        n1057 = call-dynamic "Write Channel.vi"("error in (no error)"=w2261, "Channel.lvclass"=w2263, "Acquisition in"=w2288) -> ("error out"=w2280:errorcluster, "Acquisition out"=w2279:refnum<class "Acquisition.lvclass">)  [unwired: 7 in]
        n1058 = call-dynamic "Write AcquisitionD.vi"("error in (no error)"=w2280, "Acquisition.lvclass"=w2279, "S4ACS_GUI in"=w2290) -> ("error out"=w2278:errorcluster, "S4ACS_GUI out"=w2269:refnum<class "S4GUI.lvclass">)  [unwired: 7 in]
      }
      event "Copy to Input ch1": Value Change {
        n1059 = event-data() -> ()  [unwired: 1 in, 6 out]
        n1060 = call-dynamic "Read AcquisitionA.vi"("error in (no error)"=w2325, "S4ACS_GUI in"=w2326) -> ("error out"=w2321:errorcluster, "Acquisition.lvclass"=w2324:refnum<class "Acquisition.lvclass">, "S4ACS_GUI out"=w2293:refnum<class "S4GUI.lvclass">)  [unwired: 7 in]
        n1061 = call-dynamic "Read Channel.vi"("error in (no error)"=w2321, "Acquisition in"=w2324) -> ("error out"=w2320:errorcluster, "Channel.lvclass"=w2323:refnum<class "Channel.lvclass">)  [unwired: 7 in, 1 out]
        n1062 = call-dynamic "Read Interface.vi"("error in (no error)"=w2320, "Channel in"=w2323) -> ("error out"=w2319:errorcluster, "Interface.lvclass"=w2322:refnum<class "Interface.lvclass">)  [unwired: 7 in, 1 out]
        n1063 = call-dynamic "Get CCD_Config.vi"("error in (no error)"=w2319, "Interface in"=w2322) -> ("error out"=w2316:errorcluster, "output cluster"=w2315:T24)  [unwired: 7 in, 1 out]
        n1064 = Unbundle By Name(w2315) -> ("INITIAL_LINE"=w2314:u16, "INITIAL_COLUMN"=w2313:u16, "FINAL_LINE"=w2312:u16, "FINAL_COLUMN"=w2311:u16, "VBIN"=w2310:u16, "HBIN"=w2309:u16, "PREAMP"=w2308:u8, "EM_GAIN"=w2307:u16, "READOUT_RATE"=w2306:u8, "SHUTTER_OPENING_TIME"=w2305:u16, "SHUTTER_CLOSING_TIME"=w2304:u16, "VERTICAL_SHIFT_SPEED"=w2303:u8, "READ_MODE"=w2302:u8, "VERTICAL_CLOCK_VOLTAGE"=w2301:u8, "AD_CHANNEL"=w2300:u32, "SHUTTER_MODE"=w2299:u8, "SHUTTER_TTL"=w2298:u8, "TRIGGER_MODE"=w2297:u8, "FRAME_TRANSFER"=w2296:bool, "ACQUISITION_MODE"=w2295:u8, "EM_MODE"=w2294:u8)
        n1065 = local read "Input Cluster"() -> (w2318:T6)
        n1066 = Bundle By Name(cluster=w2318, "Parameters.Image \nInitial Line"=w2314, "Parameters.Image\nInitial Column"=w2313, "Parameters.Image\nFinal Line"=w2312, "Parameters.Image\nFInal Column"=w2311, "Parameters.Vertical\nBinning"=w2310, "Parameters.Horizontal\nBinning"=w2309, "Parameters.Pre-amplification\nGain"=w2308, "Parameters.CCD\nEM Gain"=w2307, "Parameters.Readout\nRate"=w2306, "Parameters.Shutter\nOpenning Time"=w2305, "Parameters.Shutter\nClosing Time"=w2304, "Parameters.Vertical\nShift Speed"=w2303, "Parameters.Read\nMode"=w2302, "Parameters.Vertical\nClock Voltage"=w2301, "Parameters.A/D \nChannel"=w2300, "Parameters.Shutter\nMode"=w2299, "Parameters.Shutter\nTTL"=w2298, "Parameters.Trigger\nMode"=w2297, "Parameters.Frame\nTransfer"=w2296, "Parameters.Acquisition\nMode"=w2295, "Parameters.CCD \nEM Mode"=w2294) -> (w2317:T6)
        n1067 = local write "Input Cluster"(w2317) -> ()
      }
      event "Copy to Input ch2": Value Change {
        n1068 = event-data() -> ()  [unwired: 1 in, 6 out]
        n1069 = call "Read AcquisitionB.vi"("error in (no error)"=w2359, "S4ACS_GUI in"=w2360) -> ("error out"=w2355:errorcluster, "Acquisition.lvclass"=w2358:refnum<class "Acquisition.lvclass">, "S4ACS_GUI out"=w2327:refnum<class "S4GUI.lvclass">)  [unwired: 7 in]
        n1070 = call-dynamic "Read Channel.vi"("error in (no error)"=w2355, "Acquisition in"=w2358) -> ("error out"=w2354:errorcluster, "Channel.lvclass"=w2357:refnum<class "Channel.lvclass">)  [unwired: 7 in, 1 out]
        n1071 = call-dynamic "Read Interface.vi"("error in (no error)"=w2354, "Channel in"=w2357) -> ("error out"=w2353:errorcluster, "Interface.lvclass"=w2356:refnum<class "Interface.lvclass">)  [unwired: 7 in, 1 out]
        n1072 = call-dynamic "Get CCD_Config.vi"("error in (no error)"=w2353, "Interface in"=w2356) -> ("error out"=w2350:errorcluster, "output cluster"=w2349:T24)  [unwired: 7 in, 1 out]
        n1073 = Unbundle By Name(w2349) -> ("INITIAL_LINE"=w2348:u16, "INITIAL_COLUMN"=w2347:u16, "FINAL_LINE"=w2346:u16, "FINAL_COLUMN"=w2345:u16, "VBIN"=w2344:u16, "HBIN"=w2343:u16, "PREAMP"=w2342:u8, "EM_GAIN"=w2341:u16, "READOUT_RATE"=w2340:u8, "SHUTTER_OPENING_TIME"=w2339:u16, "SHUTTER_CLOSING_TIME"=w2338:u16, "VERTICAL_SHIFT_SPEED"=w2337:u8, "READ_MODE"=w2336:u8, "VERTICAL_CLOCK_VOLTAGE"=w2335:u8, "AD_CHANNEL"=w2334:u32, "SHUTTER_MODE"=w2333:u8, "SHUTTER_TTL"=w2332:u8, "TRIGGER_MODE"=w2331:u8, "FRAME_TRANSFER"=w2330:bool, "ACQUISITION_MODE"=w2329:u8, "EM_MODE"=w2328:u8)
        n1074 = local read "Input Cluster"() -> (w2352:T6)
        n1075 = Bundle By Name(cluster=w2352, "Parameters.Image \nInitial Line"=w2348, "Parameters.Image\nInitial Column"=w2347, "Parameters.Image\nFinal Line"=w2346, "Parameters.Image\nFInal Column"=w2345, "Parameters.Vertical\nBinning"=w2344, "Parameters.Horizontal\nBinning"=w2343, "Parameters.Pre-amplification\nGain"=w2342, "Parameters.CCD\nEM Gain"=w2341, "Parameters.Readout\nRate"=w2340, "Parameters.Shutter\nOpenning Time"=w2339, "Parameters.Shutter\nClosing Time"=w2338, "Parameters.Vertical\nShift Speed"=w2337, "Parameters.Read\nMode"=w2336, "Parameters.Vertical\nClock Voltage"=w2335, "Parameters.A/D \nChannel"=w2334, "Parameters.Shutter\nMode"=w2333, "Parameters.Shutter\nTTL"=w2332, "Parameters.Trigger\nMode"=w2331, "Parameters.Frame\nTransfer"=w2330, "Parameters.Acquisition\nMode"=w2329, "Parameters.CCD \nEM Mode"=w2328) -> (w2351:T6)
        n1076 = local write "Input Cluster"(w2351) -> ()
      }
      event "Copy to Input ch3": Value Change {
        n1077 = event-data() -> ()  [unwired: 1 in, 6 out]
        n1078 = call-dynamic "Read AcquisitionC.vi"("error in (no error)"=w2393, "S4ACS_GUI in"=w2394) -> ("error out"=w2389:errorcluster, "Acquisition.lvclass"=w2392:refnum<class "Acquisition.lvclass">, "S4ACS_GUI out"=w2361:refnum<class "S4GUI.lvclass">)  [unwired: 7 in]
        n1079 = call-dynamic "Read Channel.vi"("error in (no error)"=w2389, "Acquisition in"=w2392) -> ("error out"=w2388:errorcluster, "Channel.lvclass"=w2391:refnum<class "Channel.lvclass">)  [unwired: 7 in, 1 out]
        n1080 = call-dynamic "Read Interface.vi"("error in (no error)"=w2388, "Channel in"=w2391) -> ("error out"=w2387:errorcluster, "Interface.lvclass"=w2390:refnum<class "Interface.lvclass">)  [unwired: 7 in, 1 out]
        n1081 = call-dynamic "Get CCD_Config.vi"("error in (no error)"=w2387, "Interface in"=w2390) -> ("error out"=w2384:errorcluster, "output cluster"=w2383:T24)  [unwired: 7 in, 1 out]
        n1082 = Unbundle By Name(w2383) -> ("INITIAL_LINE"=w2382:u16, "INITIAL_COLUMN"=w2381:u16, "FINAL_LINE"=w2380:u16, "FINAL_COLUMN"=w2379:u16, "VBIN"=w2378:u16, "HBIN"=w2377:u16, "PREAMP"=w2376:u8, "EM_GAIN"=w2375:u16, "READOUT_RATE"=w2374:u8, "SHUTTER_OPENING_TIME"=w2373:u16, "SHUTTER_CLOSING_TIME"=w2372:u16, "VERTICAL_SHIFT_SPEED"=w2371:u8, "READ_MODE"=w2370:u8, "VERTICAL_CLOCK_VOLTAGE"=w2369:u8, "AD_CHANNEL"=w2368:u32, "SHUTTER_MODE"=w2367:u8, "SHUTTER_TTL"=w2366:u8, "TRIGGER_MODE"=w2365:u8, "FRAME_TRANSFER"=w2364:bool, "ACQUISITION_MODE"=w2363:u8, "EM_MODE"=w2362:u8)
        n1083 = local read "Input Cluster"() -> (w2386:T6)
        n1084 = Bundle By Name(cluster=w2386, "Parameters.Image \nInitial Line"=w2382, "Parameters.Image\nInitial Column"=w2381, "Parameters.Image\nFinal Line"=w2380, "Parameters.Image\nFInal Column"=w2379, "Parameters.Vertical\nBinning"=w2378, "Parameters.Horizontal\nBinning"=w2377, "Parameters.Pre-amplification\nGain"=w2376, "Parameters.CCD\nEM Gain"=w2375, "Parameters.Readout\nRate"=w2374, "Parameters.Shutter\nOpenning Time"=w2373, "Parameters.Shutter\nClosing Time"=w2372, "Parameters.Vertical\nShift Speed"=w2371, "Parameters.Read\nMode"=w2370, "Parameters.Vertical\nClock Voltage"=w2369, "Parameters.A/D \nChannel"=w2368, "Parameters.Shutter\nMode"=w2367, "Parameters.Shutter\nTTL"=w2366, "Parameters.Trigger\nMode"=w2365, "Parameters.Frame\nTransfer"=w2364, "Parameters.Acquisition\nMode"=w2363, "Parameters.CCD \nEM Mode"=w2362) -> (w2385:T6)
        n1085 = local write "Input Cluster"(w2385) -> ()
      }
      event "Copy to Input ch4": Value Change {
        n1086 = event-data() -> ()  [unwired: 1 in, 6 out]
        n1087 = Unbundle By Name(w2397) -> ("Parameters"=w2396:T23)
        n1088 = Unbundle By Name(w2396) -> ("CCD \nEM Mode"=→"CCD \nEM Mode":u8)
        n1089 = property on="CCD \nEM Mode" class="DigNum (strict)" props=["Value"]() -> ()  [unwired: 2 in, 3 out]
        n1090 = call-dynamic "Read AcquisitionD.vi"("error in (no error)"=w2430, "S4ACS_GUI in"=w2431) -> ("error out"=w2426:errorcluster, "Acquisition.lvclass"=w2429:refnum<class "Acquisition.lvclass">, "S4ACS_GUI out"=w2398:refnum<class "S4GUI.lvclass">)  [unwired: 7 in]
        n1091 = call-dynamic "Read Channel.vi"("error in (no error)"=w2426, "Acquisition in"=w2429) -> ("error out"=w2425:errorcluster, "Channel.lvclass"=w2428:refnum<class "Channel.lvclass">)  [unwired: 7 in, 1 out]
        n1092 = call-dynamic "Read Interface.vi"("error in (no error)"=w2425, "Channel in"=w2428) -> ("error out"=w2424:errorcluster, "Interface.lvclass"=w2427:refnum<class "Interface.lvclass">)  [unwired: 7 in, 1 out]
